vi "set channel.vi"(8 "error in":errorcluster, 10 "TBM channel in":refnum<class "TBM channel.lvclass">, 11 "bin datalogger configuration in":refnum<class "Binary datalogger configuration.lvclass">) -> (0 "error out":errorcluster, 3 "bin datalogger configuration out":refnum<class "Binary datalogger configuration.lvclass">)   [LabVIEW 2013, in "Binary datalogger configuration.lvclass"]
uses:
  Binary datalogger configuration.lvclass
  <vilib>/NI/Tag Bus Module Framework/channel/TBM channel.lvclass
  <vilib>/NI/Tag Bus/tag/tag descriptor.lvclass/tag descriptor.ctl
  Binary datalogger configuration.lvclass/Binary datalogger configuration.ctl
  <vilib>/NI/Tag Bus/tag/tag descriptor.lvclass
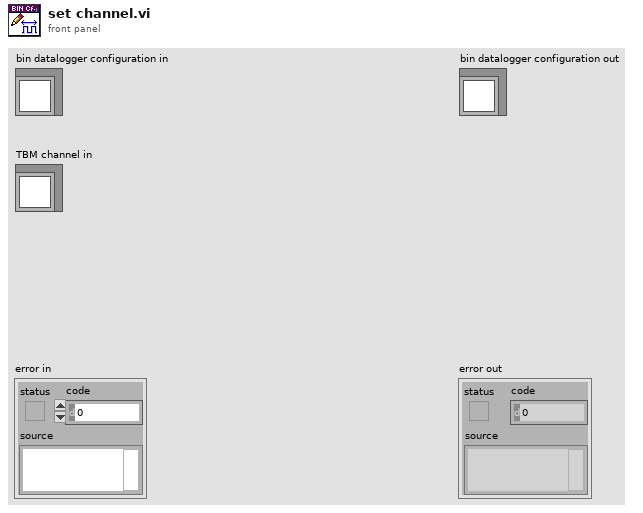
[diagram p1: front panel]
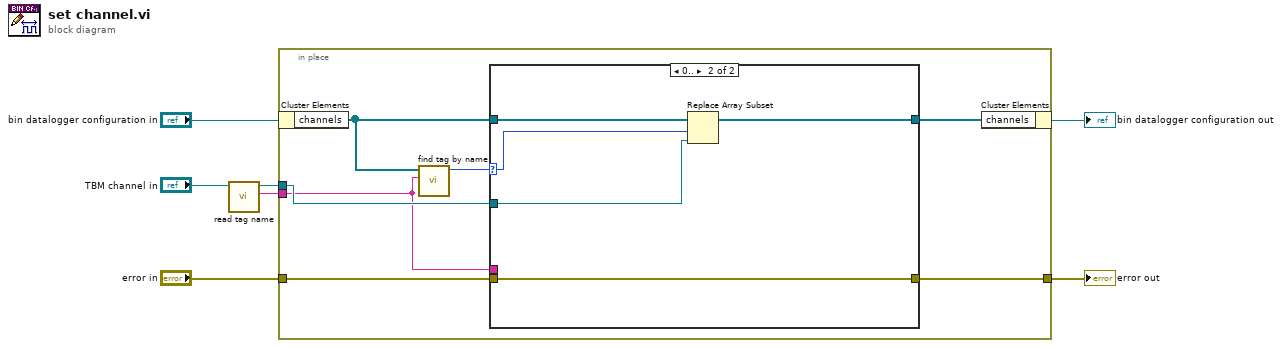
[diagram p0: block diagram]
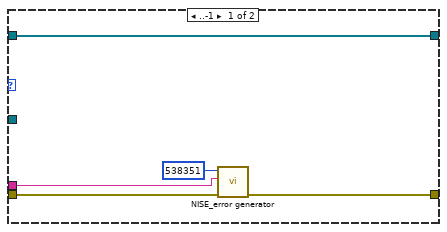
[diagram p2: hidden frame]
diagram:
  n1 = call <vilib>:"read tag name.vi"("system tag in"="TBM channel in") -> ("name"=w6:string, "system tag out"=w7:refnum<class "TBM channel.lvclass">)  [unwired: 8 in, 1 out]
  n2 = in-place {
    in-place-border: [w13] -> w3
    in-place-border: "error in" -> [w11]
    in-place-border: w7 -> [w10]
    in-place-border: w6 -> [w8]
    n3 = in-place-cluster #1("bin datalogger configuration in") -> ("channels"=w14:refnum<class "TBM channel.lvclass">[])
    n4 = call <vilib>:"find tag by name.vi"("name"=w8, "tags in"=w14) -> ("index"=w9:i32)  [unwired: 9 in]
    n5 = case shown="0.." w9 {
      selector: w9 -> [_ w20]
      tunnel: w14 -> [w17 w23]
      tunnel: [w18 w24] -> w13
      tunnel: [w17 w22] -> w12
      tunnel: w11 -> [w16 w24]
      tunnel: w10 -> [_ w21]
      tunnel: w8 -> [w15 _]
      frame ..-1 {
        n6 = call <vilib>:"NISE_error generator.vi"("error in"=w16, "append error message"=w15, "error code (0)"=538351) -> ("error out"=w18:errorcluster)  [unwired: 6 in]
      }
      frame 0.. {
        n7 = Replace Array Subset(array=w23, new element=w21, index=w20) -> (w22:refnum<class "TBM channel.lvclass">[])
      }
    }
    n8 = in-place-cluster #1("channels"=w12) -> (→"bin datalogger configuration out":refnum<class "Binary datalogger configuration.lvclass">)
  }
  "error out" <- w3
